vi "Save Data.vi"(0 "VISA resource name":refnum<visa-resource-name>, 1 "Dedicated Reading Buffer (1: Reading Buffer 1)":i32(ring)=1 items=["Reading Buffer 1"=1, "Reading Buffer 2"=2], 2 "File Name (/usb1/mybuffer)":string="/usb1/mybuffer", 5 "Source Measure Unit Channel (0: Channel A)":i32(ring) items=["Channel A", "Channel B"], 7 "Data Type (0: Dedicated Reading Buffer)":i32(ring) items=["Dedicated Reading Buffer ", "User Defined Buffer"], 9 "Memory Type (0: Nonvolatile Memory)":i32(ring) items=["Nonvolatile Memory ", "USB Flash Drive"], 11 "error in (no error)":errorcluster, 12 "User Defined Reading Buffer":string, 13 "File Format (0: CSV)":i32(ring) items=["CSV", "XML"]) -> (4 "VISA resource name out":refnum<visa-resource-name>, 15 "error out":errorcluster)   [LabVIEW 2020, in "Keithley 2600 Series.lvlib"]
doc: "Saves data to nonvolatile memory or USB flash driver."
uses:
  <instrlib>/Keithley 2600 Series/Keithley 2600 Series.lvlib
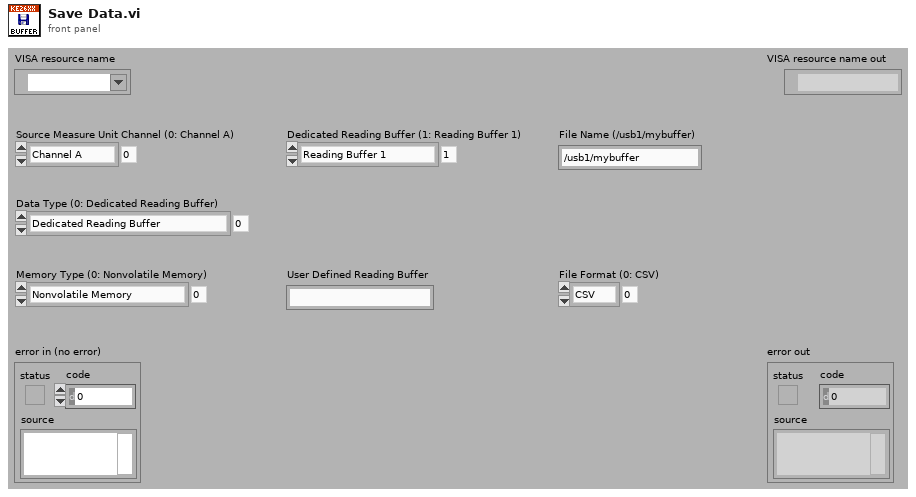
[diagram p1: front panel]
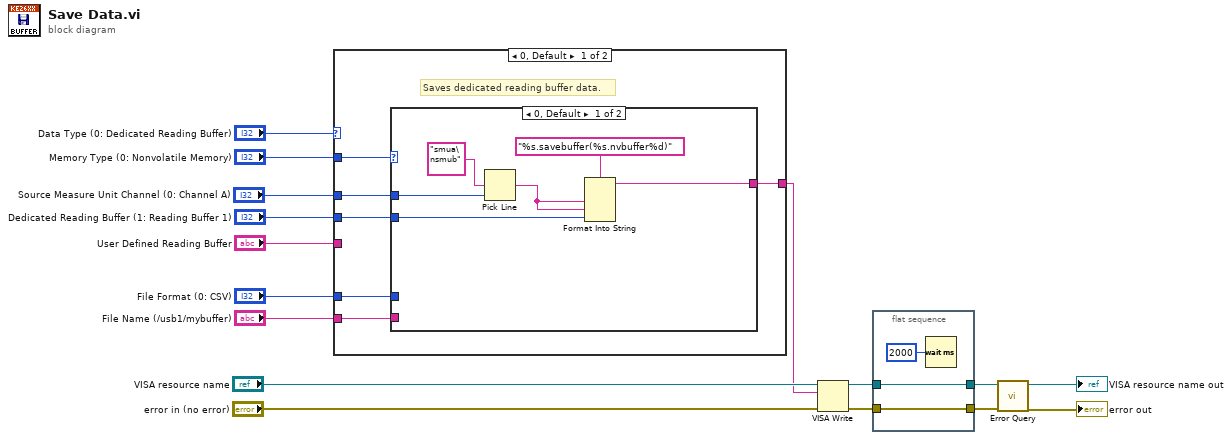
[diagram p0: block diagram]
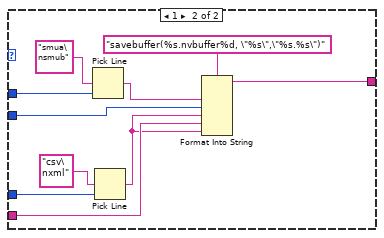
[diagram p2: hidden frame]
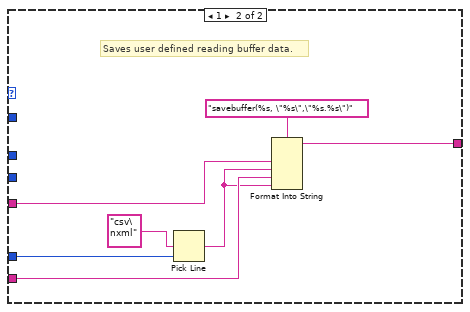
[diagram p3: hidden frame]
diagram:
  n1 = case shown="0, Default" "Data Type (0: Dedicated Reading Buffer)" {
    tunnel: "Source Measure Unit Channel (0: Channel A)" -> [w21 _]
    tunnel: "Dedicated Reading Buffer (1: Reading Buffer 1)" -> [w22 _]
    tunnel: [w20 w40] -> w5
    tunnel: "User Defined Reading Buffer" -> [_ w43]
    tunnel: "Memory Type (0: Nonvolatile Memory)" -> [w19 _]
    tunnel: "File Format (0: CSV)" -> [w18 w41]
    tunnel: "File Name (/usb1/mybuffer)" -> [w17 w42]
    frame 0, Default {
      # "Saves dedicated reading buffer data."
      n2 = case shown="0, Default" w19 {
        tunnel: w22 -> [w24 w33]
        tunnel: w21 -> [w25 w37]
        tunnel: [w23 w35] -> w20
        tunnel: w18 -> [_ w31]
        tunnel: w17 -> [_ w30]
        frame 0, Default {
          n3 = Pick Line(multi-line string="smua\nsmub", line index=w25) -> (output string=w26:string)  [unwired: 1 in]
          n4 = Format Into String(format string="%s.savebuffer(%s.nvbuffer%d)", w26, w26, w24) -> (resulting string=w23:string)  [unwired: 2 in, 1 out]
        }
        frame 1 {
          n5 = Pick Line(multi-line string="smua\nsmub", line index=w37) -> (output string=w34:string)  [unwired: 1 in]
          n6 = Pick Line(multi-line string="csv\nxml", line index=w31) -> (output string=w29:string)  [unwired: 1 in]
          n7 = Format Into String(format string="savebuffer(%s.nvbuffer%d, \"%s\",\"%s.%s\")", w34, w33, w29, w30, w29) -> (resulting string=w35:string)  [unwired: 2 in, 1 out]
        }
      }
    }
    frame 1 {
      # "Saves user defined reading buffer data."
      n8 = Pick Line(multi-line string="csv\nxml", line index=w41) -> (output string=w39:string)  [unwired: 1 in]
      n9 = Format Into String(format string="savebuffer(%s, \"%s\",\"%s.%s\")", w43, w39, w42, w39) -> (resulting string=w40:string)  [unwired: 2 in, 1 out]
    }
  }
  n10 = VISA Write(VISA resource name="VISA resource name", write buffer=w5, error in (no error)="error in (no error)") -> (VISA resource name out=w4:refnum<visa-resource-name>, error out=w3:errorcluster)  [unwired: 1 out]
  n11 = flat-sequence {
    tunnel: w4 -> [w48]
    tunnel: w3 -> [w47]
    tunnel: [w48] -> w2
    tunnel: [w47] -> w1
    frame #0 {
      n12 = Wait (ms)(milliseconds to wait=u32 2000) -> ()  [unwired: 1 out]
    }
  }
  n13 = call <instrlib>:"Error Query.vi"("error in (no error)"=w1, "VISA resource name"=w2) -> ("error out"=→"error out":errorcluster, "VISA resource name out"=→"VISA resource name out":refnum<visa-resource-name>)  [unwired: 6 in, 2 out]
